vi "Get Switches.vi"(8 "error in (no error)":errorcluster, 11 "MC switch refnum in":refnum<k24>) -> (0 "error out":errorcluster, 2 "switch states":bool[](array[boolean]), 3 "MC switch refnum out":refnum<k24>)   [LabVIEW 2019, in "Minicircuit RF Switch Box.lvlib"]
doc: "Get the states of all switches in the switch matrix. If no swich are connected at a position, the state will always be false.\n\n<b>switch states:</b> the array of the switch state. The sate of A is at the index 0 and H at the index 7."
uses:
  <instrlib>/Minicircuit RF Switch Box/Minicircuit RF Switch Box.lvlib
  C:/Program Files (x86)/National Instruments/LabVIEW 2019/instr.lib/Minicircuit RF Switch Box/mcl_RF_Switch_Controller_NET45.dll
  mcl_RF_Switch_Controller_NET45.dll
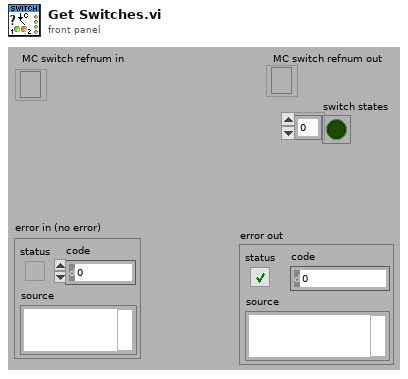
[diagram p1: front panel]
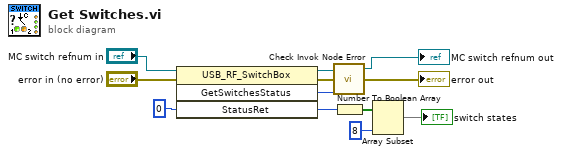
[diagram p0: block diagram]
diagram:
  n1 = invoke class="USB_RF_SwitchBox" method="GetSwitchesStatus"(reference="MC switch refnum in", error in="error in (no error)", "StatusRet"=0) -> (reference out=w10:refnum<k24>, error out=w9:errorcluster, "GetSwitchesStatus"=w8:i32, "StatusRet"=w4:i32)  [unwired: 1 in]
  n2 = call <instrlib>:"Check Invok Node Error.vi"("Connect"=w8, "error in (no error)"=w9, "MC switch refnum in"=w10) -> ("error out"=→"error out":errorcluster, "MC switch refnum out"=→"MC switch refnum out":refnum<k24>)  [unwired: 1 in]
  n3 = Number To Boolean Array(number=w4) -> (Boolean array=w3:bool[])
  n4 = Array Subset(array=w3, length=8) -> (→"switch states":bool[])  [unwired: 1 in]
